vi "GE 5565PIORC.PIO.Read In-Place (U32).vi"(7 "byte order (big-endian)":T1(ring), 8 "error in (no error)":errorcluster, 9 "data in":u32, 10 "offset":u32, 11 "GE 5565PIORC in":refnum<class "GE 5565PIORC.lvclass">) -> (0 "error out":errorcluster, 1 "data out":u32, 3 "GE 5565PIORC out":refnum<class "GE 5565PIORC.lvclass">)   [LabVIEW 2017, in "GE 5565PIORC.lvclass"]
doc: "Reads from the specified <B>offset</B> and places the contents into <B>data</B>."
uses:
  GE 5565PIORC.lvclass
  <vilib>/Instr/_visa.llb/VISA Register Access Address Space.ctl
  GE 5565PIORC.lvclass/GE 5565PIORC.ctl
  GE 5565PIORC.VISA.Move In-Place.String (U8).vi
  GE 5565PIORC.VISA.Return Handler.vi
  <vilib>/Utility/error.llb/Error Cluster From Error Code.vi
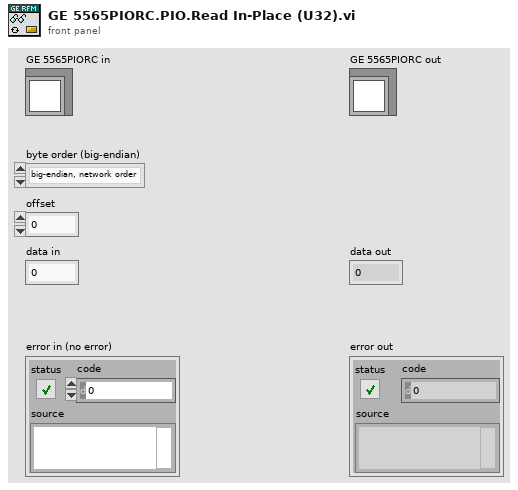
[diagram p1: front panel]
types:
  T1 = enum16{"big-endian, network order", "native, host order", "little-endian"}
  T2 = typedef "VISA Register Access Address Space.ctl" = u16
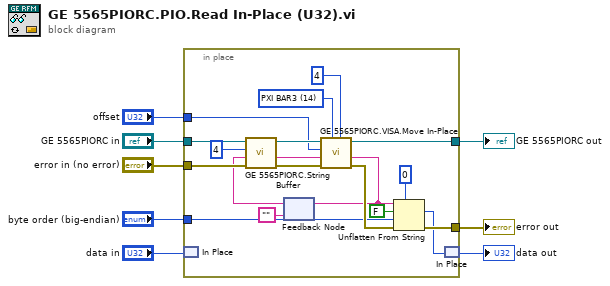
[diagram p0: block diagram]
diagram:
  n1 = in-place {
    in-place-border: "error in (no error)" -> [w20]
    in-place-border: [w27] -> w7
    in-place-border: "GE 5565PIORC in" -> [w21]
    in-place-border: "offset" -> [w13]
    in-place-border: "byte order (big-endian)" -> [w15]
    in-place-border: [w24] -> w3
    w25 = T2 14 items=["VXI/VME A16"=1, "VXI/VME A24"=2, "VXI/VME A32"=3, "VXI/VME A64"=4, "PXI Memory Allocations"=9, "PXI Configuration"=10, "PXI BAR0"=11, "PXI BAR1"=12, "PXI BAR2"=13, "PXI BAR3"=14, "PXI BAR4"=15, "PXI BAR5"=16] ("address space")
    n2 = in-place-match #1("data in") -> ()  [unwired: 1 out]
    n3 = feedback #2("" ("data out")) -> (w16:string)
    n4 = call "GE 5565PIORC.String Buffer.vi"("error in (no error)"=w20, "string buffer in"=w16, "minimum size"=4, "GE 5565PIORC in"=w21) -> ("error out"=w19:errorcluster, "string buffer out"=w18:string, "GE 5565PIORC out"=w22:refnum<class "GE 5565PIORC.lvclass">)  [unwired: 5 in]
    n5 = call-poly "GE 5565PIORC.VISA.Move In-Place.vi"("count (-1: all)"=4, "address space"=w25, "error in (no error)"=w19, "data in"=w18, "offset"=w13, "GE 5565PIORC in"=w22) -> ("error out"=w23:errorcluster, "data out"=w17:string, "GE 5565PIORC out"=w24:refnum<class "GE 5565PIORC.lvclass">)  [unwired: 3 in]
    n6 = feedback-in #2(w17) -> ()
    n7 = Unflatten From String(type=u32 0, binary string=w17, data includes array or string size? (T)=FALSE, byte order (0:big-endian, network order)=w15, error in (no error)=w23) -> (value=w12:u32, error out=w27:errorcluster)  [unwired: 1 out]
    n8 = in-place-match #1(w12) -> (→"data out":u32)
  }
  "GE 5565PIORC out" <- w3
  "error out" <- w7
